vi "Area.vi"(10 "Blade Length (m/s)":dbl) -> (2 "Area (m^2)":dbl)   [LabVIEW 2018]
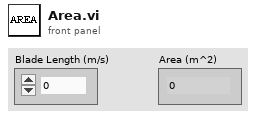
[diagram p1: front panel]
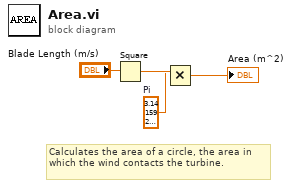
[diagram p0: block diagram]
diagram:
  w3 = 3.141592653589793  # Pi
  # "Calculates the area of a circle, the area in which the wind contacts the turbine."
  n1 = Square(x="Blade Length (m/s)") -> (x^2=w4:dbl)
  n2 = Multiply(x=w4, y=w3) -> (x*y=→"Area (m^2)":dbl)
